vi "debug wrapper.vi"(7 "Attribute":T1=7 items=["Plain White"=7, "Bold White"=15, "Bold Blue"=9, "Bold Green"=10, "Bold Red"=12], 10 "Add to log file? (T)":bool, 11 "Message":string) -> ()   [LabVIEW 2014, in "Scriptable Model Interface Engine.lvlib"]
uses:
  Engine/Scriptable Model Interface Engine.lvlib
  <vilib>/NI Veristand/Custom Device Tools/Custom Device Utility Library/Custom Device Utility Library.lvlib
  <vilib>/NI Veristand/Custom Device Tools/Custom Device Utility Library/RT Debug String Color Spec.ctl
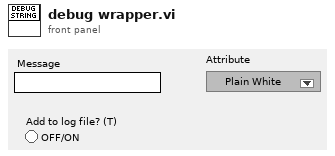
[diagram p1: front panel]
types:
  T1 = typedef "Custom Device Utility Library.lvlib/RT Debug String Color Spec.ctl" = u16
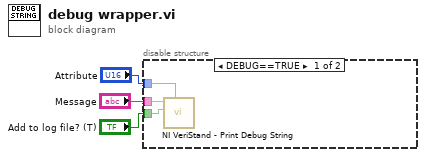
[diagram p0: block diagram]
diagram:
  n1 = disable-structure shown="DEBUG==TRUE" {
    disable-tunnel: "Attribute" -> [w6 _]
    disable-tunnel: "Add to log file? (T)" -> [w5 _]
    disable-tunnel: "Message" -> [w4 _]
    frame condition #0 {
      n2 = call <vilib>:"NI VeriStand - Print Debug String.vi"("Attribute"=w6, "Add to log file? (T)"=w5, "Message"=w4) -> ()  [unwired: 8 in, 1 out]
    }
    frame condition #1 (active) {
    }
  }
